vi "Parse ChipID.vi"(8 "error in (no error)":errorcluster, 11 "String":string) -> (0 "error out":errorcluster, 3 "ChipID":u8)   [LabVIEW 2018, in "Config Parser BML.lvlib" / "Config Parser BML.lvclass"]
uses:
  Config Parser BML.lvclass
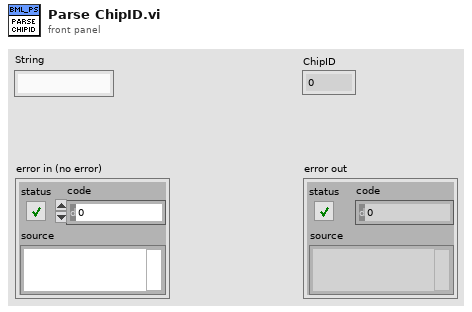
[diagram p1: front panel]
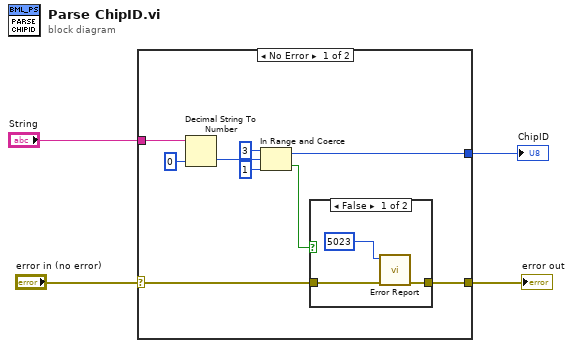
[diagram p0: block diagram]
diagram:
  n1 = case shown="No Error" "error in (no error)" {
    selector: "error in (no error)" -> [w7 w18]
    tunnel: "String" -> [w13 _]
    tunnel: [w6 w18] -> w2
    tunnel: [w5 _] -> w1
    frame No Error {
      n2 = Decimal String To Number(string=w13, default (0L)=u8 0 ("default (0 I32)")) -> (number=w11:u8)  [unwired: 1 in, 1 out]
      n3 = In Range and Coerce(upper limit=u8 3, x=w11, lower limit=u8 1) -> (coerced(x)=w5:u8, In Range?=w8:bool)
      n4 = case shown="False" w8 {
        tunnel: w7 -> [w15 w17]
        tunnel: [w14 w17] -> w6
        frame False {
          n5 = call "Error Report.vi"("error in (no error)"=w15, "Error Code"=i16 5023) -> ("error out"=w14:errorcluster)  [unwired: 9 in]
        }
        frame True {
        }
      }
    }
    frame Error {
    }
  }
  "error out" <- w2
  "ChipID" <- w1
